vi "try to reach vi server.vi"(8 "error in":errorcluster, 11 "port":u32) -> (0 "error out":errorcluster, 2 "connected":bool, 3 "Application out":refnum<vi>)   [LabVIEW 2013]
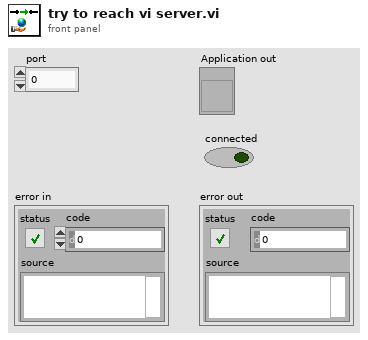
[diagram p1: front panel]
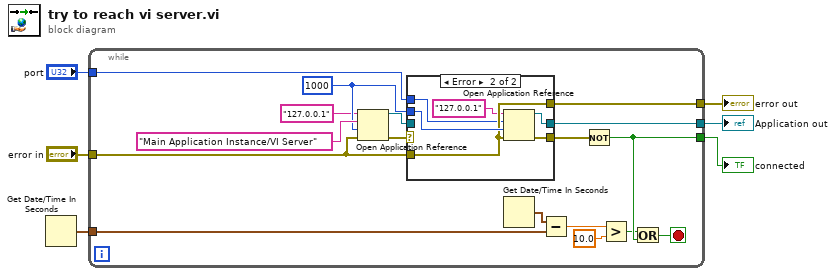
[diagram p0: block diagram]
diagram:
  n1 = Get Date/Time In Seconds() -> (seconds since 1Jan1904=w6:timestamp)
  n2 = while {
    tunnel: "port" -> [w20]
    tunnel: "error in" -> [w19]
    tunnel: [w17] -> w3
    tunnel: [w12] -> w4
    tunnel: [w16] -> w5
    tunnel: w6 -> [w13]
    stop <- w11 stop-if-true
    w18 = 1000 ("timeout ms (60000)")
    n3 = Open Application Reference(8:w19, 9:w18, 10:"Main Application Instance/VI Server", 11:"127.0.0.1" ("machine name (\"\":  open local reference)")) -> (0:w22:errorcluster, 3:w21:refnum<vi>)
    n4 = case shown="Error" w22 {
      selector: w22 -> [w24 _]
      tunnel: w21 -> [w25 _]
      tunnel: w20 -> [_ w26]
      tunnel: [w25 w29] -> w17
      tunnel: [w24 w31] -> w7
      tunnel: w19 -> [_ w28]
      tunnel: w18 -> [_ w30]
      tunnel: [w24 w28] -> w16
      frame No Error {
      }
      frame Error {
        n5 = Open Application Reference(8:w28, 9:w30, 10:w26, 11:"127.0.0.1" ("machine name (\"\":  open local reference)")) -> (0:w31:errorcluster, 3:w29:refnum<vi>)
      }
    }
    n6 = Get Date/Time In Seconds() -> (seconds since 1Jan1904=w14:timestamp)
    n7 = Subtract(x=w14, y=w13) -> (x-y=w8:dbl)
    n8 = Not(x=w7) -> (.not. x?=w12:bool)
    n9 = Greater?(x=w8, y=10.0) -> (0:w10:bool)
    n10 = Or(x=w10, y=w12) -> (x .or. y?=w11:bool)
  }
  "error out" <- w5
  "connected" <- w4
  "Application out" <- w3
